vi "Sparse_Uncorrelated.vi"(8 "error in (no error)":errorcluster caption="entrée d'erreur (pas d'erreur)", 11 "make_sparse_uncorrelated":T2={"n_samples"=100, "n_features"=10, "random_state"=-1, "Returns"="X"} {"random_state" min=-1; "n_samples" min=1}) -> (0 "error out":errorcluster, 3 "Data":T1)   [LabVIEW 2020]
doc: "Generate a random regression problem with sparse uncorrelated design :\n\nX ~ N(0, 1)\ny(X) = X[:, 0] + 2 * X[:, 1] - 2 * X[:, 2] - 1.5 * X[:, 3]\n\nOnly the first 4 features are informative. The remaining features are useless.\n\n\nParameters :\n\n- n_samples : int, optional (default=100)\nThe number of samples.\n\n- n_features : int, optional (default=10)\nThe number of features.\n\n- random_state : int, RandomState instance, default=None=-1\nDetermines random number generation for dataset creation. Pass an int for reproducible output across multiple function calls. See Glossary.\n\nReturns :\n\n- X : array of shape [n_samples, n_features]\nThe input samples.\n\n- y : array of shape [n_samples]\nThe output values."
uses:
  Sparse_Uncorrelated.lvclass
panel:
  out "Sparse_Uncorrelated.lvclass":refnum<class "Sparse_Uncorrelated.lvclass">
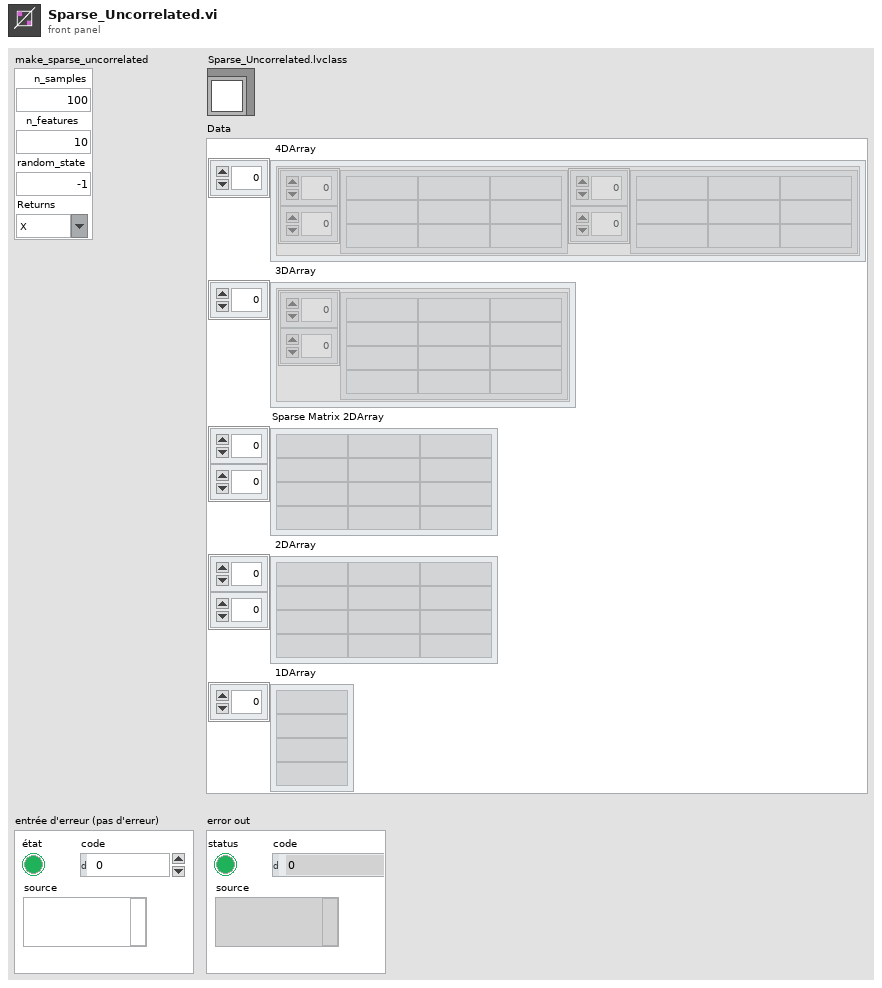
[diagram p1: front panel]
types:
  T1 = cluster{" 4DArray":cluster{"1":string[][], "2":string[][]}[], " 3DArray":cluster{"Tableau":string[][]}[], "Sparse Matrix 2DArray":string[][], " 2DArray":string[][], " 1DArray":string[]}
  T2 = cluster{"n_samples":u32, "n_features":i32, "random_state":i32, "Returns":string}
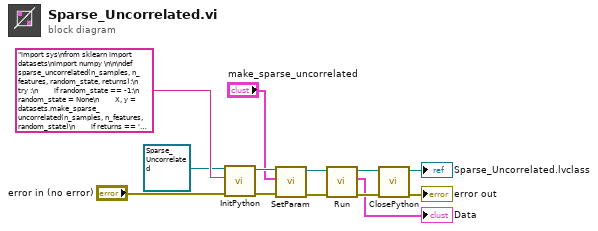
[diagram p0: block diagram]
diagram:
  n1 = call-dynamic "InitPython.vi"("error in (no error)"="error in (no error)", "Python Instruction"="import sys\nfrom sklearn import datasets\nimport numpy \n\n\ndef sparse_uncorrelated(n_samples, n_features, random_state, returns):\n    try :\n        if random_state == -1:\n            random_state = None\n        X, y = datasets.make_sparse_uncorrelated(n_samples, n_features, random_state)\n        if returns == 'X':\n            dataX = X.tolist()\n            return str(dataX)\n        else:\n            datay = y.tolist()\n            return str(datay)\n    except:\n        erreur = sys.exc_info()\n        typerr = u\"%s\" % (erreur[0])\n        typerr = typerr[typerr.find(\"'\")+1:typerr.rfind(\"'\")]\n        msgerr = u\"%s\" % (erreur[1])\n        message = str('/!\\\\ {0} : {1}'. format(typerr,msgerr))\n        return message", "Scikit-learn en entrée"=refnum<class "Sparse_Uncorrelated.lvclass"> refnum ("Sparse_Uncorrelated.lvclass")) -> ("error out"=w8:errorcluster, "Scikit-learn en sortie"=w10:refnum<class "Sparse_Uncorrelated.lvclass">)  [unwired: 7 in]
  n2 = call-dynamic "SetParam.vi"("error in (no error)"=w8, "make_sparse_uncorrelated"="make_sparse_uncorrelated", "Sparse_Uncorrelated.lvclass"=w10) -> ("error out"=w7:errorcluster, "Sparse_Uncorrelated.lvclass"=w4:refnum<class "Sparse_Uncorrelated.lvclass">)  [unwired: 7 in]
  n3 = call-dynamic "Run.vi"("error in (no error)"=w7, "Sparse_Uncorrelated.lvclass"=w4) -> ("error out"=w5:errorcluster, "Data"=→"Data":T1, "Sparse_Uncorrelated.lvclass"=w6:refnum<class "Sparse_Uncorrelated.lvclass">)  [unwired: 7 in]
  n4 = call-dynamic "ClosePython.vi"("error in (no error)"=w5, "Scikit-learn en entrée"=w6) -> ("error out"=→"error out":errorcluster, "Scikit-learn en sortie"=→"Sparse_Uncorrelated.lvclass":refnum<class "Sparse_Uncorrelated.lvclass">)  [unwired: 8 in]
